vi "GetThermAlarmTemperature.vi"(8 "error in":errorcluster, 10 "ThermAlarm number":T1=1 items=["ThermAlarm 1"=1, "ThermAlarm 2"=2, "ThermAlarm 3"=3, "ThermAlarm 4"=4], 11 "VISA resource name":refnum<visa-resource-name>) -> (0 "error out":errorcluster, 1 "ThermAlarm temperature":i32, 2 "ThermAlarm temperature string":string, 3 "VISA resource name out":refnum<visa-resource-name>)   [LabVIEW 2023, in "Thermotron 8800.lvlib"]
doc: "THAT\nCommand name: Send Therm-Alarm temperature\nCommand type: Variable\nDescription: The query command asks the 8800 for the current Therm-Alarm “n” temperature reading. The 8800 sends the temperature value as an integer.\nSyntax: THATn\nWhere n is a Therm-Alarm number (1 through 4).\nData type: Integer\nQuery example: THAT1?\n8800 response: 65 (The current temperature reading for Therm-Alarm 1 is 65.)"
uses:
  Thermotron 8800.lvlib
  Private/ThermAlarmNumber.ctl
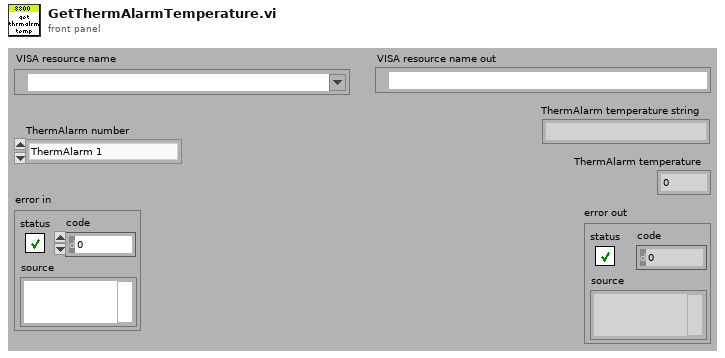
[diagram p1: front panel]
types:
  T1 = typedef "Thermotron 8800.lvlib/ThermAlarmNumber.ctl" = u16
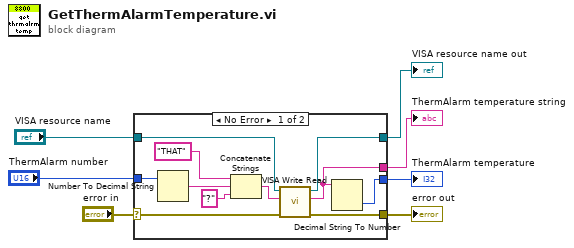
[diagram p0: block diagram]
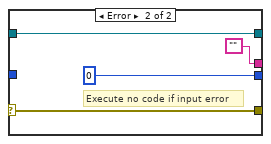
[diagram p2: hidden frame]
diagram:
  n1 = case shown="No Error" "error in" {
    selector: "error in" -> [w12 w22]
    tunnel: [w11 w22] -> w4
    tunnel: "VISA resource name" -> [w14 w21]
    tunnel: [w13 w21] -> w5
    tunnel: "ThermAlarm number" -> [w10 _]
    tunnel: [w9 ""] -> w2
    tunnel: [w8 0] -> w1
    frame No Error {
      n2 = Number To Decimal String(number=w10) -> (decimal integer string=w18:string)  [unwired: 1 in]
      n3 = Concatenate Strings("THAT" ("8800 Command"), w18, "?" ("8800 Command")) -> (w17:string)
      n4 = call "VISA Write Read.vi"("error in (no error)"=w12, "8800 Command"=w17, "VISA Refnum in"=w14) -> ("error out"=w11:errorcluster, "read buffer"=w9:string, "VISA Refnum out"=w13:refnum<visa-resource-name>)  [unwired: 6 in]
      n5 = Decimal String To Number(string=w9) -> (number=w8:i32)  [unwired: 2 in, 1 out]
    }
    frame Error {
      # "Execute no code if input error"
    }
  }
  "error out" <- w4
  "VISA resource name out" <- w5
  "ThermAlarm temperature string" <- w2
  "ThermAlarm temperature" <- w1
